vi "pulse-laser.vi"() -> ()   [LabVIEW 2014]
panel:
  in  "time_off_s":dbl=1.0 caption="Time Off [s]" format="%#_6p"
  in  "time_on_s":dbl=1.0 caption="Time On [s]" format="%#_6p"
  in  "exit":bool
  in  "start":bool
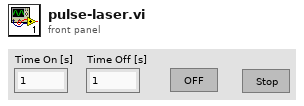
[diagram p1: front panel]
types:
  T1 = cluster{"Instruct Data":i32, "Op Code":i32, "Flags":bool[], "Comments":string, "Time":dbl}
  T2 = cluster{"Instruct Data":i32, "Op Code":i32, "Flags":bool[], "Comments":string, "Time":dbl}[]
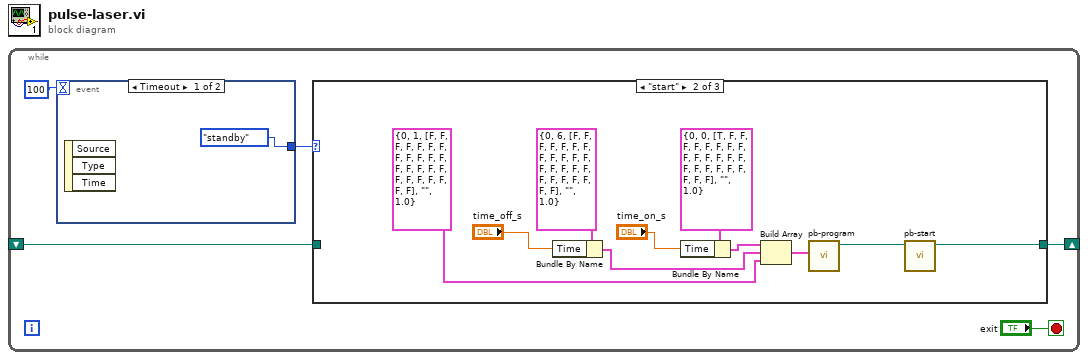
[diagram p0: block diagram]
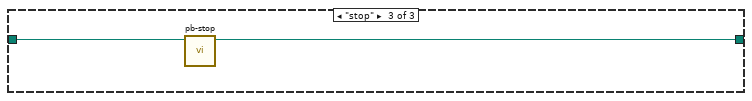
[diagram p3: hidden frame]
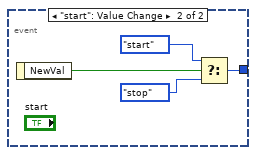
[diagram p4: hidden frame]
diagram:
  n1 = while {
    shift-right: [w4] -> _
    shift-left: _ -> [w3]
    stop <- "exit" stop-if-true
    n2 = event shown="[0] Timeout" {
      selector: _ -> [_ _]
      dyn-events: _ -> [_ _]
      timeout: 100 -> [_ _]
      tunnel: [enum16{"standby", "start", "stop"}."standby" w23] -> w2
      event Timeout {
        n3 = event-data() -> ()  [unwired: 1 in, 3 out]
      }
      event "start": Value Change {
        n4 = event-data() -> ("NewVal"=w21:bool)  [unwired: 1 in]
        n5 = Select(t=enum16{"standby", "start", "stop"}."start", s=w21, f=enum16{"standby", "start", "stop"}."stop") -> (s? t:f=w23:enum16{"standby", "start", "stop"})
      }
    }
    n6 = case shown="\"start\"" w2 {
      tunnel: [w6 w10 w17] -> w4
      tunnel: w3 -> [w6 _ w18]
      frame "standby", Default {
      }
      frame "start" {
        n7 = Bundle By Name(cluster=T1 {"Instruct Data"=0, "Op Code"=6, "Flags"=[FALSE, FALSE, FALSE, FALSE, FALSE, FALSE, FALSE, FALSE, FALSE, FALSE, FALSE, FALSE, FALSE, FALSE, FALSE, FALSE, FALSE, FALSE, FALSE, FALSE, FALSE, FALSE, FALSE, FALSE], "Comments"="", "Time"=1.0} ("PB Instruction"), "Time"="time_off_s") -> (w13:T1)
        n8 = Bundle By Name(cluster=T1 {"Instruct Data"=0, "Op Code"=0, "Flags"=[TRUE, FALSE, FALSE, FALSE, FALSE, FALSE, FALSE, FALSE, FALSE, FALSE, FALSE, FALSE, FALSE, FALSE, FALSE, FALSE, FALSE, FALSE, FALSE, FALSE, FALSE, FALSE, FALSE, FALSE], "Comments"="", "Time"=1.0} ("PB Instruction"), "Time"="time_on_s") -> (w14:T1)
        n9 = Build Array(w14, w13, T1 {"Instruct Data"=0, "Op Code"=1, "Flags"=[FALSE, FALSE, FALSE, FALSE, FALSE, FALSE, FALSE, FALSE, FALSE, FALSE, FALSE, FALSE, FALSE, FALSE, FALSE, FALSE, FALSE, FALSE, FALSE, FALSE, FALSE, FALSE, FALSE, FALSE], "Comments"="", "Time"=1.0} ("PB Instruction")) -> (w12:T2)
        n10 = call "pb-program.vi"("Commands"=w12) -> ("path out"=w11:path)  [unwired: 10 in]
        n11 = call "pb-start.vi"("path in"=w11) -> ("path out"=w10:path)  [unwired: 10 in]
      }
      frame "stop" {
        n12 = call "pb-stop.vi"("path in"=w18) -> ("path out"=w17:path)  [unwired: 9 in, 1 out]
      }
    }
  }
